vi "Project.vi"() -> ()   [LabVIEW 2015]
uses:
  <vilib>/Platform/TimedLoop/XDataNode/timing_clust.ctl
  <vilib>/Platform/TimedLoop/XDataNode/nitl_modes.ctl
  <vilib>/Platform/TimedLoop/XDataNode/wakeup.ctl
  <vilib>/DAQmx/read.llb/DAQmx Read (Counter DBL 1Chan 1Samp).vi
  <vilib>/DAQmx/read.llb/DAQmx Read (Digital Bool 1Line 1Point).vi
  <vilib>/DAQmx/write.llb/DAQmx Write (Analog DBL 1Chan 1Samp).vi
  <vilib>/DAQmx/read.llb/DAQmx Read (Analog 1D DBL NChan 1Samp).vi
  <vilib>/DAQmx/create/channels.llb/DAQmx Create Channel (AI-Voltage-Basic).vi
  <vilib>/DAQmx/create/channels.llb/DAQmx Create Channel (DI-Digital Input).vi
  <vilib>/DAQmx/create/channels.llb/DAQmx Create Channel (AO-Voltage-Basic).vi
  <vilib>/DAQmx/create/channels.llb/DAQmx Create Channel (CI-Count Edges).vi
  <vilib>/DAQmx/miscellaneous.llb/DAQmx Fill In Error Info.vi
  <vilib>/Analysis/3filter.llb/Butterworth Filter (DBL).vi
  <vilib>/Utility/file.llb/Write To Spreadsheet File (DBL).vi
  <vilib>/Platform/TimedLoop/XDataNode/XDataNode.xnode
  <vilib>/Platform/TimedLoop/XDataNode/XDNodeRunTimeDep.lvlib
  <vilib>/Analysis/NI_AALBase.lvlib
panel:
  out "Controller samp. time (s)":dbl
  out "Position Vs Time":cluster{dbl, "output":dbl}(graph)
  out "Force Vs Time":cluster{dbl, "output":dbl}(graph)
  out "Gripping Time":dbl format="%0.2f"
  out "Actual Force":dbl(slide) scale=0.0..20.0
  in  "Reset 2":bool
  in  "Desired Force":dbl(slide) min=0.0 max=13.5 scale=0.0..20.0 scale format="%#_3g"
  in  "Kd (force)":dbl=0.1 step=1.0
  in  "Ki (force)":dbl=0.5 step=2.0
  in  "Kp (force)":dbl=0.1 step=1.0
  in  "Kd (pos)":dbl=0.2 step=1.0
  in  "Ki (pos)":dbl=5.0 step=2.0
  in  "Kp (pos)":dbl=5.0 step=1.0
  out "Applied Motor Voltage":dbl
  out "Current Position":dbl(slide) scale=0.0..20.0
  out "Object Size":dbl(slide) scale=0.0..50.0
  out "Motor Position (deg.)":ext(knob) scale=0.0..360.0
  in  "Position Encoder":tag="Dev4/ctr0"
  out "Clockwise":bool
  in  "Optical Encoder":tag="Dev4/port0/line6"
  in  "Tachometer":tag="Dev4/ai4"
  in  "Current":tag="Dev4/ai0"
  in  "Voltage":tag="Dev4/ao0"
  in  "Reset":bool
  in  "Desired Position":dbl(slide) min=0.0 max=18.5 scale=0.0..20.0
  out "Motor & External Torque":cluster{dbl, dbl}(graph)
  out "Motor Acceleration (rad/s^2)":dbl(knob) scale=-50.0..50.0
  out "Motor Velocity (rad/s)":ext(knob) scale=-150.0..150.0
  out "Current Draw (amps)":dbl format="%#_2g"
  out "Current Draw":dbl(graph)
  out "Applied & Terminal Motor Voltage":cluster{dbl, "output":dbl}(graph)
  in  "File Path":path=path "\\\\uoa.auckland.ac.nz\\engdfs/home/nlob862/Desktop/705/dummy_stop_csv.csv"
  in  "?":bool
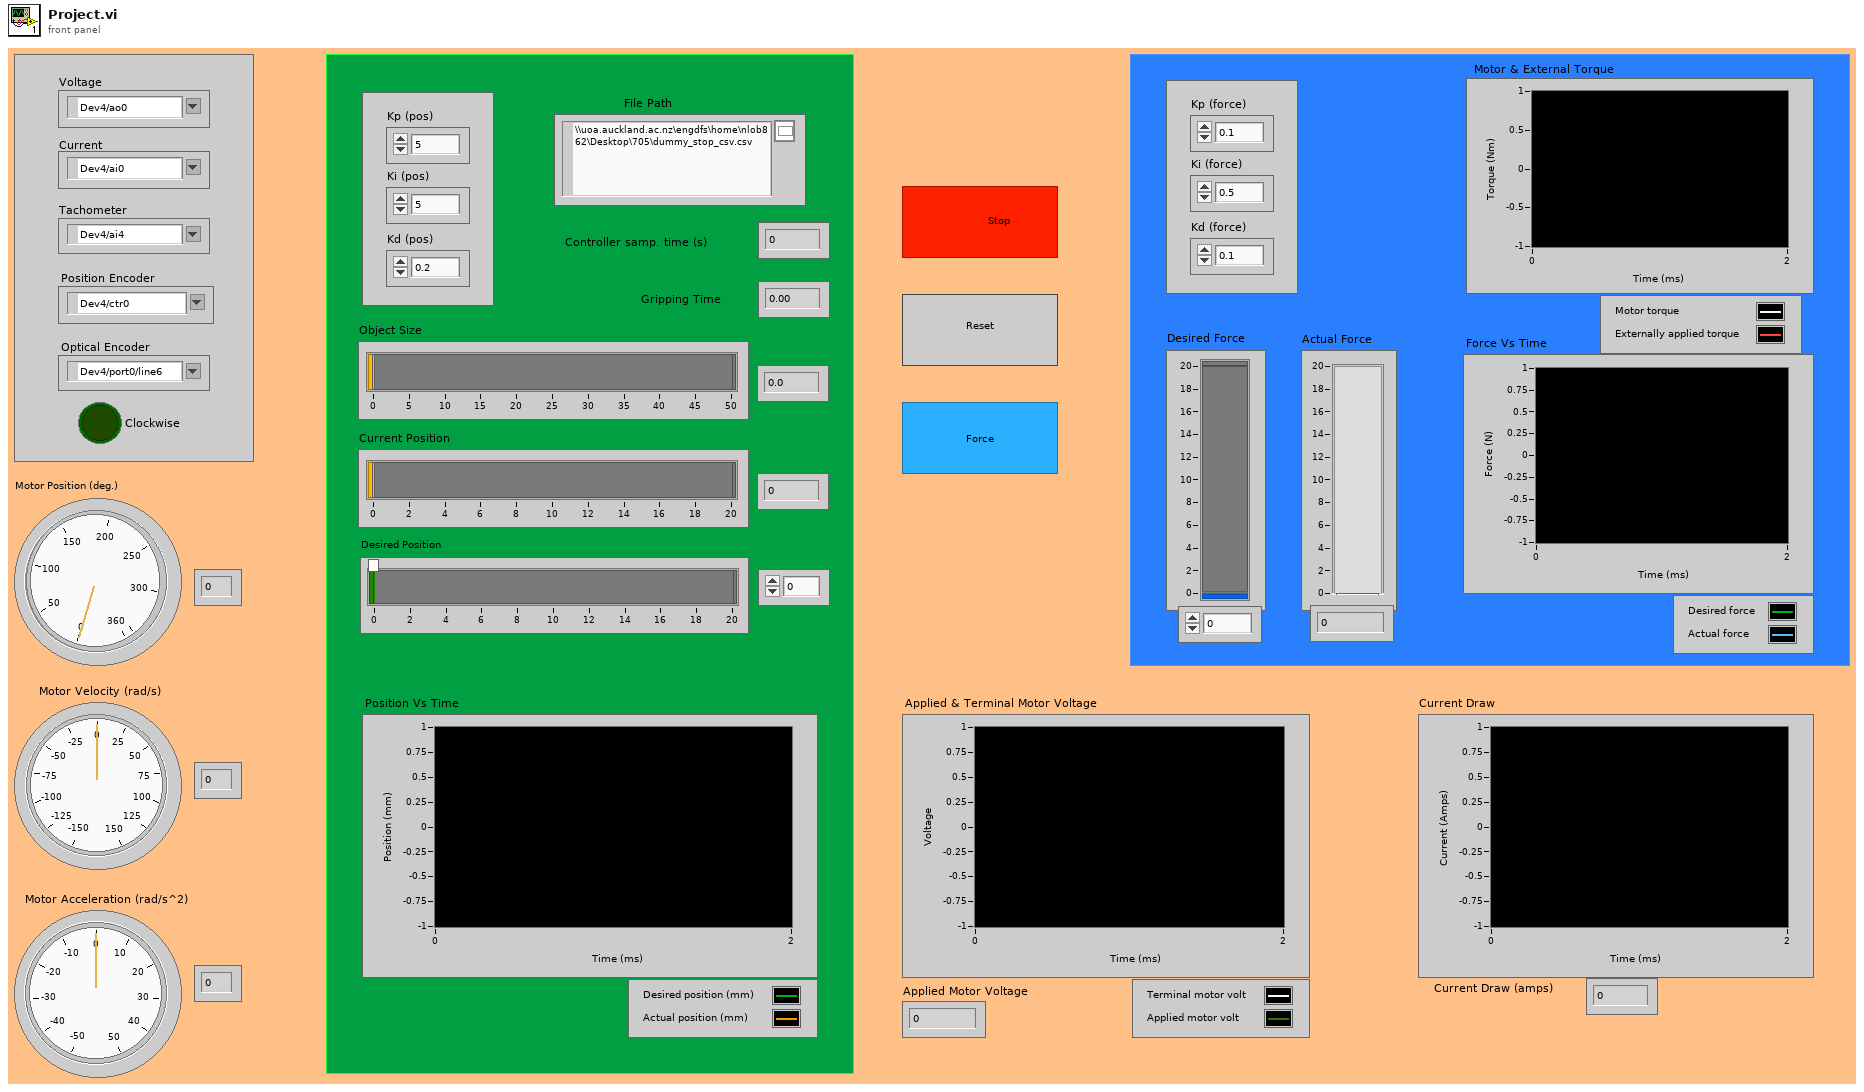
[diagram p1: front panel]
types:
  T1 = typedef "XDNodeRunTimeDep.lvlib/timing_clust.ctl" = cluster{"Expected End [f-1]":u64, "Actual End [f-1]":u64, "Finished Late? [f-1]":bool, "Expected End [i-1]":u64, "Actual End [i-1]":u64, "Finished Late? [i-1]":bool, "Expected Start [i]":u64, "Actual Start [i]":u64, "Expected Start [f]":u64, "Actual Start [f]":u64, "Source Name":string, "Structure Name":string, "Period":i64, "Deadline":i64, "Offset":i64, "Start":i64, "Priority":i32, "Timeout":i32, "Mode":T2, "Wakeup Reason":T3, "Error":errorcluster, "Source Type":string, "Secondary Source Type":string, "Global End Time":u64, "Global Start Time":u64, "Frame Duration":u64, "Iteration Duration":u64, "Assigned CPU":i32, "I/O Scan Engine Mode":u32}
  T2 = typedef "XDNodeRunTimeDep.lvlib/nitl_modes.ctl" = enum32{"No Change", "Process missed periods, maintain original phase", "Discard missed periods, maintain original phase", "Process missed periods, ignore original phase", "Discard missed periods, ignore original phase"}
  T3 = typedef "XDNodeRunTimeDep.lvlib/wakeup.ctl" = enum32{"Normal", "Aborted", "Asynchronous wakeup", "Timing source error", "Timed loop error", "Timeout"}
  T4 = cluster{"Desired Position":dbl, "Current Position":dbl}
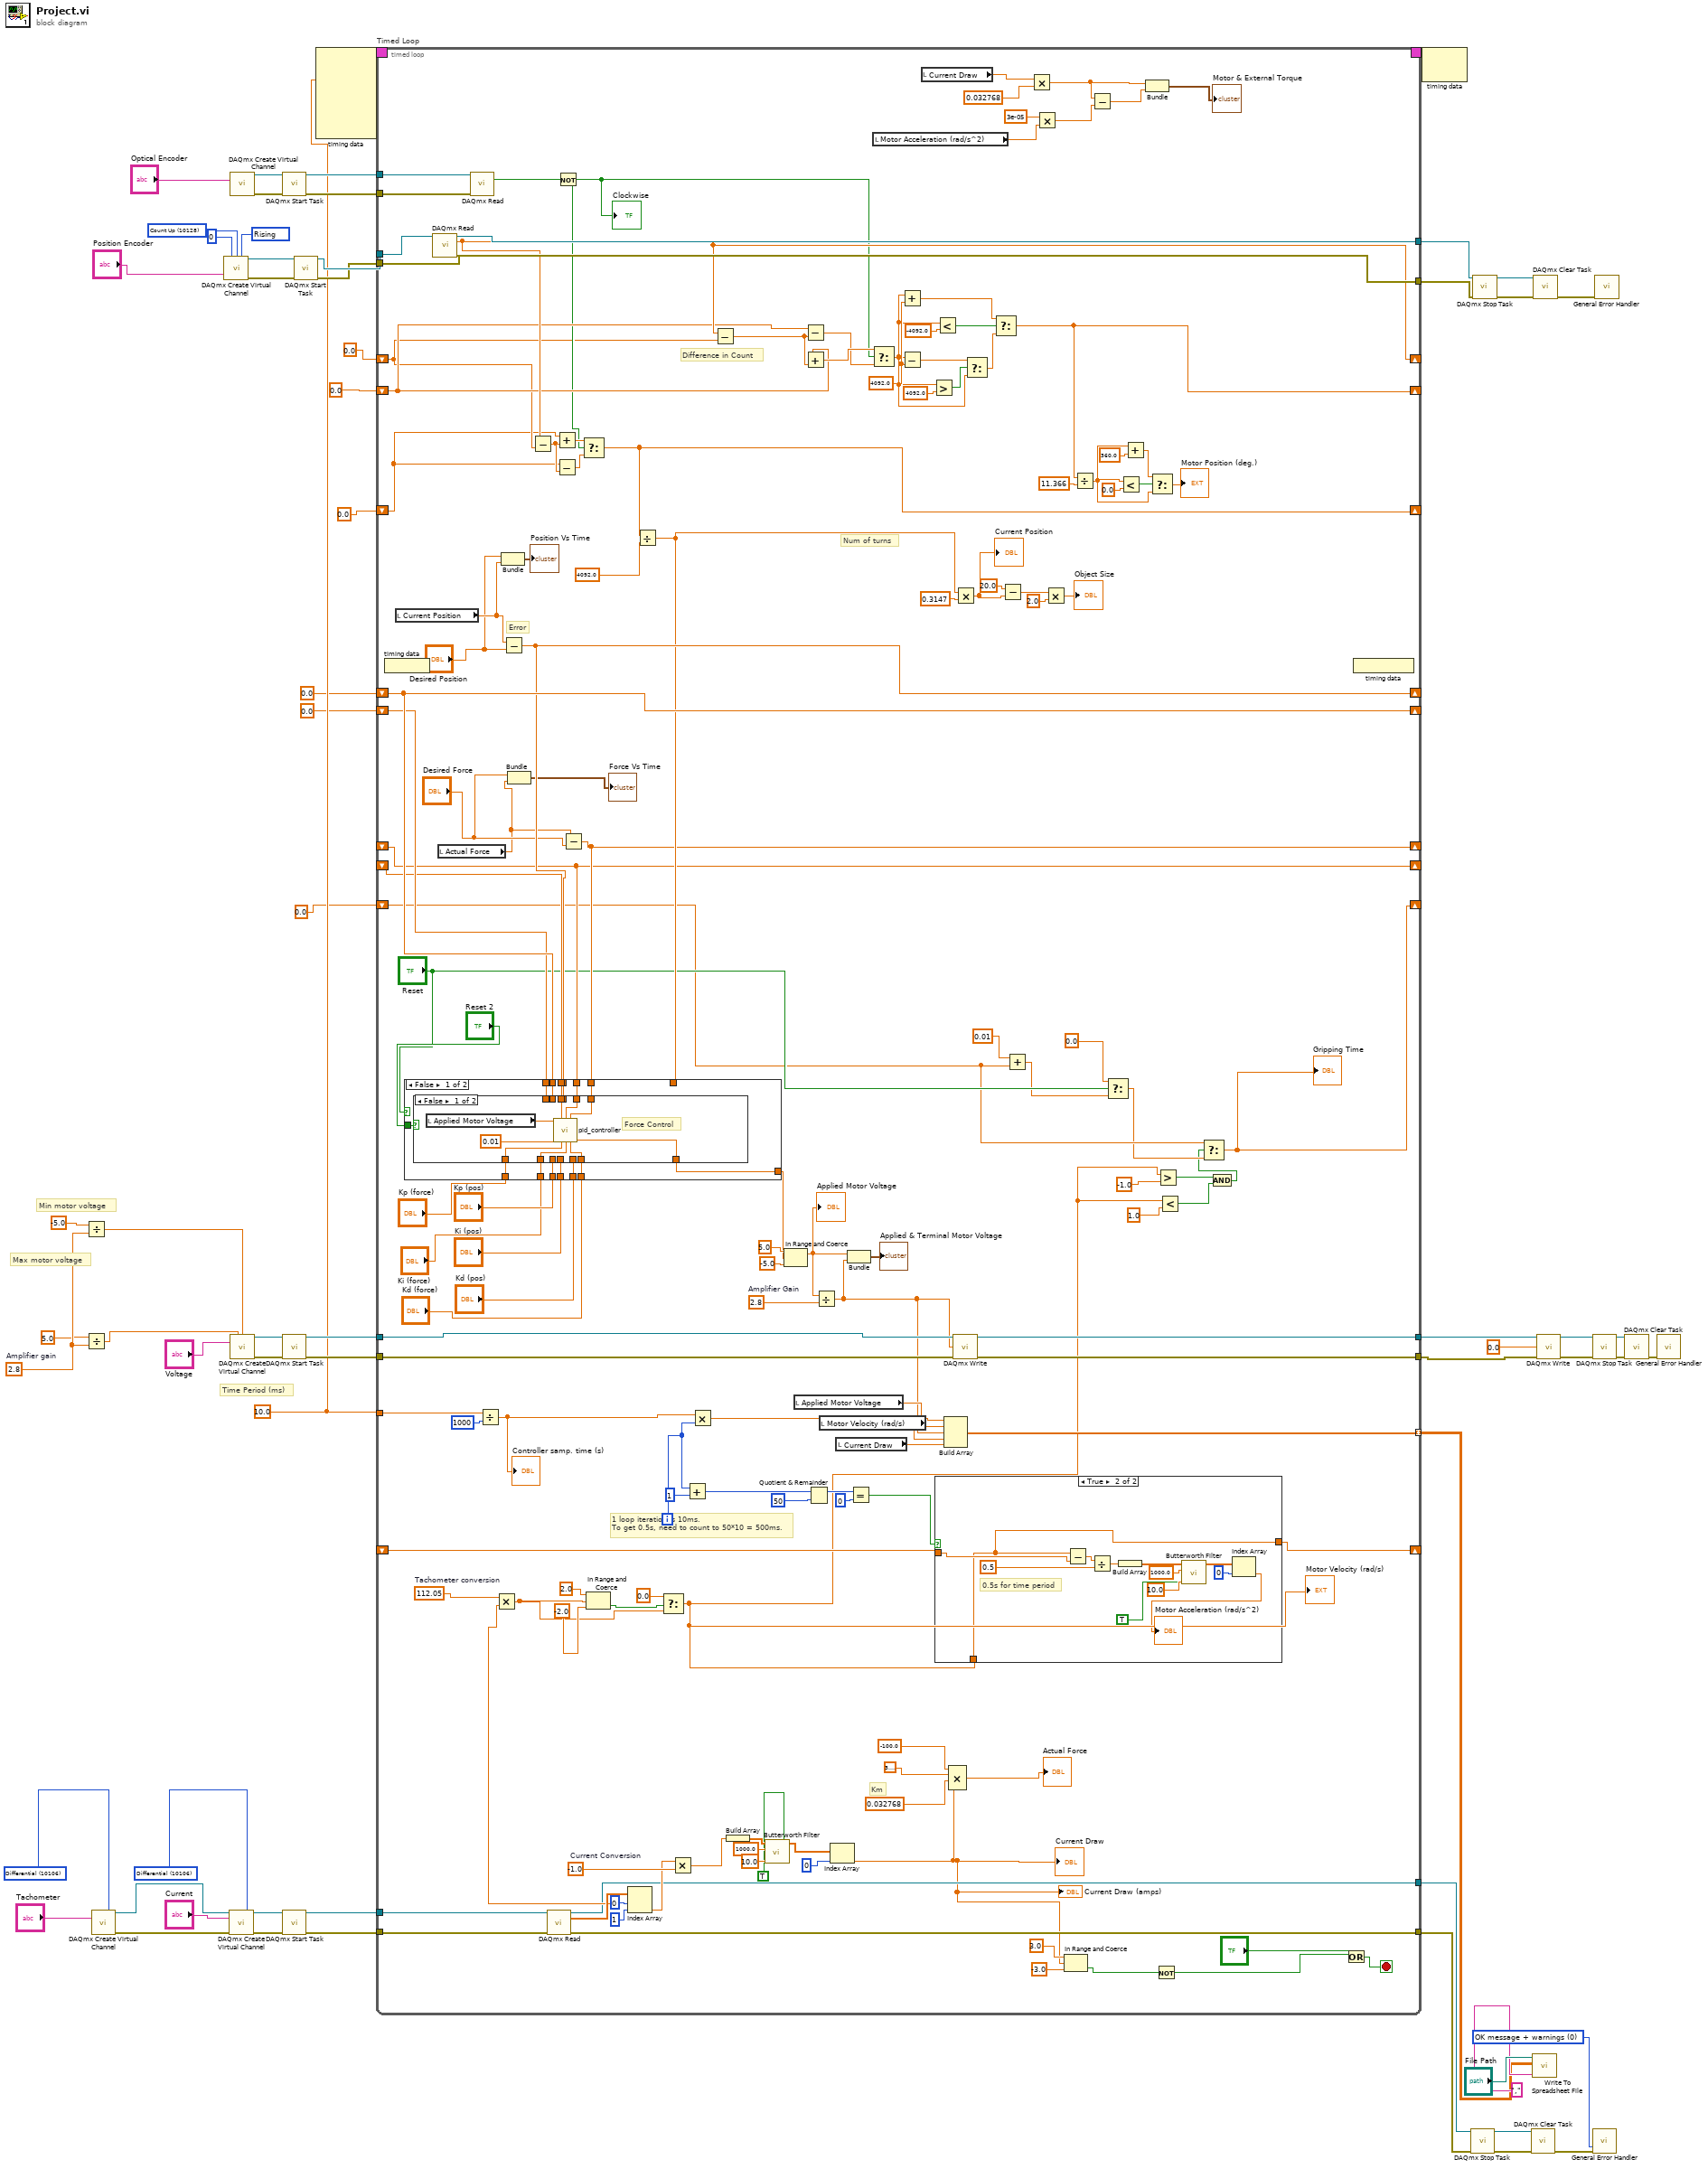
[diagram p0: block diagram]
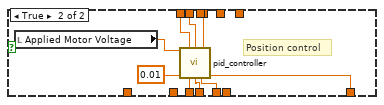
[diagram p2: hidden frame]
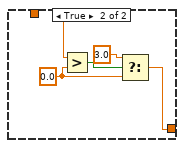
[diagram p3: hidden frame]
diagram:
  w4 = 10.0
  w8 = 10128 items=["Count Up"=10128, "Count Down"=10124, "Externally Controlled"=10326] ("count direction")
  w16 = 10280 items=["Rising"=10280, "Falling"=10171] ("edge")
  w31 = 10106 items=["Default"=-1, "RSE"=10083, "NRSE"=10078, "Differential"=10106, "Pseudodifferential"=12529] ("input terminal configuration")
  w32 = 10106 items=["Default"=-1, "RSE"=10083, "NRSE"=10078, "Differential"=10106, "Pseudodifferential"=12529] ("input terminal configuration")
  w44 = u16 0 items=["OK message + warnings"]
  w30 = 2.8  # Amplifier gain
  # "Time Period (ms)"
  # "Max motor voltage"
  # "Min motor voltage"
  n1 = Divide(x=-5.0, y=w30) -> (x/y=w49:dbl)
  n2 = Divide(x=5.0, y=w30) -> (x/y=w29:dbl)
  n3 = call-poly <vilib>:"DAQmx Create Virtual Channel.vi"("input terminal configuration"=w31, "physical channels"="Tachometer") -> ("task out"=w55:refnum<k21>, "error out"=w58:errorcluster)  [unwired: 12 in]
  n4 = call-poly <vilib>:"DAQmx Create Virtual Channel.vi"("initial count"=u32 0, "count direction"=w8, "edge"=w16, "counter"="Position Encoder") -> ("task out"=w20:refnum<k21>, "error out"=w19:errorcluster)  [unwired: 10 in]
  n5 = call-poly <vilib>:"DAQmx Create Virtual Channel.vi"("task in"=w55, "input terminal configuration"=w32, "physical channels"="Current", "error in"=w58) -> ("task out"=w56:refnum<k21>, "error out"=w57:errorcluster)  [unwired: 10 in]
  n6 = call-poly <vilib>:"DAQmx Create Virtual Channel.vi"("lines"="Optical Encoder") -> ("task out"=w27:refnum<k21>, "error out"=w25:errorcluster)  [unwired: 13 in]
  n7 = call-poly <vilib>:"DAQmx Create Virtual Channel.vi"("maximum value"=w29, "minimum value"=w49, "physical channels"="Voltage") -> ("task out"=w62:refnum<k21>, "error out"=w61:errorcluster)  [unwired: 11 in]
  n8 = call <vilib>:"DAQmx Start Task.vi"("task/channels in"=w27, "error in"=w25) -> ("task out"=w26:refnum<k21>, "error out"=w24:errorcluster)  [unwired: 12 in]
  n9 = call <vilib>:"DAQmx Start Task.vi"("task/channels in"=w62, "error in"=w61) -> ("task out"=w51:refnum<k21>, "error out"=w50:errorcluster)  [unwired: 12 in]
  n10 = call <vilib>:"DAQmx Start Task.vi"("task/channels in"=w56, "error in"=w57) -> ("task out"=w54:refnum<k21>, "error out"=w53:errorcluster)  [unwired: 12 in]
  n11 = call <vilib>:"DAQmx Start Task.vi"("task/channels in"=w20, "error in"=w19) -> ("task out"=w18:refnum<k21>, "error out"=w14:errorcluster)  [unwired: 12 in]
  n12 = node-c288(w4) -> (w64:T1)  [unwired: 5 in]
  n13 = timed-loop "Timed Loop" {
    timing: w64 -> [_]
    timing-out: [_] -> w63
    tunnel: w54 -> [w210]
    tunnel: w53 -> [w209]
    tunnel: w51 -> [w194]
    tunnel: w50 -> [w193]
    tunnel: [w197] -> w40
    tunnel: [w196] -> w39
    tunnel: w4 -> [w195]
    tunnel: [w191] -> w36
    tunnel: [w192] -> w38
    tunnel: [w199] -> w33 mode=indexing
    tunnel: w26 -> [w188]
    tunnel: w24 -> [w187]
    shift-right: [w182] -> _
    shift-left: _ -> [w183]
    tunnel: w18 -> [w169]
    tunnel: w14 -> [w168]
    tunnel: [w167] -> w10
    tunnel: [w166] -> w9
    shift-right: [w143] -> _
    shift-left: 0.0 -> [w139]
    shift-right: [w151] -> _
    shift-left: 0.0 -> [w142]
    shift-right: [w137] -> _
    shift-left: 0.0 -> [w138]
    shift-right: [w117] -> _
    shift-left: 0.0 -> [w122]
    shift-right: [w122] -> _
    shift-left: 0.0 -> [w121]
    shift-right: [w111] -> _
    shift-left: _ -> [w110]
    shift-right: [w110] -> _
    shift-left: _ -> [w109]
    shift-right: [w96] -> _
    shift-left: 0.0 -> [w97]
    i -> [w185]
    stop <- w76 stop-if-true
    w156 = 4092.0
    w208 = -1.0  # Current Conversion
    w207 = 112.05  # Tachometer conversion
    w198 = 2.8  # Amplifier Gain
    # "Num of turns"
    # "Km"
    # "Error"
    # "Difference in Count"
    # "1 loop iteration is 10ms.\nTo get 0.5s, need to count to 50*10 = 500ms."
    n14 = node-c288() -> ()  [unwired: 1 in]
    n15 = local read "Current Position"() -> (w86:dbl)
    n16 = call-poly <vilib>:"DAQmx Read.vi"("task/channels in"=w169, "error in"=w168) -> ("task out"=w167:refnum<k21>, "data"=w143:dbl, "error out"=w166:errorcluster)  [unwired: 11 in]
    n17 = local read "Actual Force"() -> (w65:dbl)
    n18 = call-poly <vilib>:"DAQmx Read.vi"("task/channels in"=w188, "error in"=w187) -> ("data"=w186:bool)  [unwired: 11 in, 2 out]
    n19 = Divide(x=w195, y=1000) -> (x/y=w126:dbl)
    "Controller samp. time (s)" <- w126
    n20 = Bundle("Desired Position"="Desired Position", "Current Position"=w86) -> (→"Position Vs Time":T4)  [unwired: 1 in]
    n21 = Subtract(x=w86, y="Desired Position") -> (x-y=w117:dbl)
    n22 = Bundle("Desired Force"="Desired Force", "Actual Force"=w65) -> (→"Force Vs Time":cluster{"Desired Force":dbl, "Actual Force":dbl})  [unwired: 1 in]
    n23 = Subtract(x=w143, y=w139) -> (x-y=w141:dbl)
    n24 = call-poly <vilib>:"DAQmx Read.vi"("task/channels in"=w210, "error in"=w209) -> ("task out"=w196:refnum<k21>, "data"=w206:dbl[], "error out"=w197:errorcluster)  [unwired: 11 in]
    n25 = Add(x=w138, y=w141) -> (x+y=w145:dbl)
    n26 = Subtract(x=w138, y=w141) -> (x-y=w144:dbl)
    n27 = Not(x=w186) -> (.not. x?=w140:bool)
    "Clockwise" <- w140
    n28 = Subtract(x=w65, y="Desired Force") -> (x-y=w111:dbl)
    n29 = Select(t=w145, s=w140, f=w144) -> (s? t:f=w137:dbl)
    n30 = Index Array(array=w206, index #1=0, index #2=1) -> (element #1=w203:dbl, element #2=w202:dbl)
    n31 = Multiply(x=w207, y=w203) -> (x*y=w172:dbl)
    n32 = In Range and Coerce(upper limit=2.0, x=w172, lower limit=-2.0) -> (In Range?=w174:bool)  [unwired: 1 out]
    n33 = Divide(x=w137, y=4092.0) -> (x/y=w116:dbl)
    n34 = case shown="False" "Reset" {
      tunnel: w116 -> [_ w244]
      tunnel: [w218 w243] -> w123
      tunnel: w117 -> [w222 _]
      tunnel: w122 -> [w223 _]
      tunnel: w121 -> [w224 _]
      tunnel: "Kp (pos)" -> [w221 _]
      tunnel: "Ki (pos)" -> [w220 _]
      tunnel: "Kd (pos)" -> [w219 _]
      tunnel: "Reset 2" -> [w217 _]
      tunnel: "Kp (force)" -> [w216 _]
      tunnel: "Ki (force)" -> [w215 _]
      tunnel: "Kd (force)" -> [w214 _]
      tunnel: w111 -> [w213 _]
      tunnel: w110 -> [w212 _]
      tunnel: w109 -> [w211 _]
      frame False {
        n35 = case shown="False" w217 {
          tunnel: w224 -> [_ w242]
          tunnel: w223 -> [_ w241]
          tunnel: w222 -> [_ w240]
          tunnel: w221 -> [_ w237]
          tunnel: w220 -> [_ w236]
          tunnel: w219 -> [_ w235]
          tunnel: [w225 w234] -> w218
          tunnel: w216 -> [w231 _]
          tunnel: w215 -> [w230 _]
          tunnel: w214 -> [w229 _]
          tunnel: w213 -> [w228 _]
          tunnel: w212 -> [w227 _]
          tunnel: w211 -> [w226 _]
          frame False {
            # "Force Control"
            n36 = local read "Applied Motor Voltage"() -> (w232:dbl)
            n37 = call "pid_controller.vi"("Motor Voltage 1 Sample Ago"=w232, "Error 2 Samples Ago"=w226, "Error 1 Sample Ago"=w227, "Error (Current)"=w228, "Time (dt)"=0.01, "Kp"=w231, "Ki"=w230, "Kd"=w229) -> ("Motor Voltage for Next Sample"=w225:dbl)  [unwired: 7 in]
          }
          frame True {
            # "Position control"
            n38 = local read "Applied Motor Voltage"() -> (w239:dbl)
            n39 = call "pid_controller.vi"("Motor Voltage 1 Sample Ago"=w239, "Error 2 Samples Ago"=w242, "Error 1 Sample Ago"=w241, "Error (Current)"=w240, "Time (dt)"=0.01, "Kp"=w237, "Ki"=w236, "Kd"=w235) -> ("Motor Voltage for Next Sample"=w234:dbl)  [unwired: 7 in]
          }
        }
      }
      frame True {
        w245 = 0.0
        n40 = Greater?(x=w244, y=w245) -> (0:w246:bool)
        n41 = Select(t=3.0, s=w246, f=w245) -> (s? t:f=w243:dbl)
      }
    }
    n42 = Select(t=0.0, s=w174, f=w172) -> (s? t:f=w92:dbl)
    "Motor Velocity (rad/s)" <- w92
    n43 = Multiply(x=w202, y=w208) -> (x*y=w80:dbl)
    n44 = Add(x=w185, y=1) -> (x+y=w179:i32)
    n45 = Multiply(x=w126, y=w185) -> (x*y=w200:dbl)
    n46 = Subtract(x=w143, y=w139) -> (x-y=w165:dbl)
    n47 = Build Array(w80) -> (w103:dbl[])
    n48 = call-poly <vilib>:"Butterworth Filter.vi"("init/cont (init:F)"=TRUE, "low cutoff freq: fl"=10.0, "sampling freq: fs"=1000.0, "X"=w103) -> ("Filtered X"=w74:dbl[])  [unwired: 4 in, 1 out]
    n49 = In Range and Coerce(upper limit=5.0, x=w123, lower limit=-5.0 ("upper limit")) -> (coerced(x)=w108:dbl)  [unwired: 1 out]
    "Applied Motor Voltage" <- w108
    n50 = local read "Applied Motor Voltage"() -> (w129:dbl)
    n51 = Subtract(x=w142, y=w165) -> (x-y=w163:dbl)
    n52 = Add(x=w142, y=w165) -> (x+y=w164:dbl)
    n53 = Quotient & Remainder(x=w179, y=50) -> (x-y*floor(x/y)=w178:i32)  [unwired: 1 out]
    n54 = Divide(x=w108, y=w198) -> (x/y=w125:dbl)
    n55 = local read "Motor Velocity (rad/s)"() -> (w190:ext)
    n56 = Index Array(array=w74, index=0) -> (element=w73:dbl)
    "Current Draw" <- w73
    "Current Draw (amps)" <- w73
    n57 = local read "Current Draw"() -> (w189:dbl)
    n58 = Bundle("upper limit"=w108, w125) -> (→"Applied & Terminal Motor Voltage":cluster{"upper limit":dbl, dbl})  [unwired: 1 in]
    n59 = Equal?(x=w178, y=0) -> (x = y?=w184:bool)
    n60 = Select(t=w164, s=w140, f=w163) -> (s? t:f=w146:dbl)
    n61 = local read "Motor Acceleration (rad/s^2)"() -> (w67:dbl)
    n62 = Add(x=w146, y=w156) -> (x+y=w155:dbl)
    n63 = Subtract(x=w146, y=w156) -> (x-y=w159:dbl)
    n64 = local read "Current Draw"() -> (w171:dbl)
    n65 = Greater?(x=w146, y=4092.0) -> (0:w160:bool)
    n66 = case shown="True" w184 {
      tunnel: w92 -> [_ w259]
      tunnel: w183 -> [w248 w260]
      tunnel: [w248 w259] -> w182
      frame False {
      }
      frame True {
        # "0.5s for time period"
        n67 = Subtract(x=w259, y=w260) -> (x-y=w258:dbl)
        n68 = Divide(x=w258, y=0.5) -> (x/y=w250:dbl)
        n69 = Build Array(w250) -> (w254:dbl[])
        n70 = call-poly <vilib>:"Butterworth Filter.vi"("init/cont (init:F)"=TRUE, "low cutoff freq: fl"=10.0, "sampling freq: fs"=1000.0, "X"=w254) -> ("Filtered X"=w251:dbl[])  [unwired: 4 in, 1 out]
        n71 = Index Array(array=w251, index=0) -> (element=→"Motor Acceleration (rad/s^2)":dbl)
      }
    }
    n72 = Less?(x=w146, y=-4092.0) -> (x < y?=w157:bool)
    n73 = Build Array(w200, w129, w125, w190, w189) -> (w199:ext[])
    n74 = Compound Arithmetic op=MULTIPLY(-100.0 ("x"), 3.141592653589793, 0.032768 ("x"), w73) -> (→"Actual Force":dbl)
    n75 = call-poly <vilib>:"DAQmx Write.vi"("task/channels in"=w194, "data"=w125, "error in"=w193) -> ("task out"=w191:refnum<k21>, "error out"=w192:errorcluster)  [unwired: 10 in, 1 out]
    n76 = Multiply(x=w116, y=0.3147) -> (x*y=w130:dbl)
    "Current Position" <- w130
    n77 = Select(t=w159, s=w160, f=w146) -> (s? t:f=w158:dbl)
    n78 = Select(t=w155, s=w157, f=w158) -> (s? t:f=w151:dbl)
    n79 = Subtract(x=20.0 ("y"), y=w130) -> (x-y=w134:dbl)
    n80 = Add(x=0.01 ("y"), y=w97) -> (x+y=w100:dbl)
    n81 = Multiply(x=w171, y=0.032768) -> (x*y=w71:dbl)
    n82 = Multiply(x=3e-05, y=w67) -> (x*y=w69:dbl)
    n83 = Multiply(x=w134, y=2.0) -> (x*y=→"Object Size":dbl)
    n84 = In Range and Coerce(upper limit=3.0, x=w73, lower limit=-3.0) -> (In Range?=w79:bool)  [unwired: 1 out]
    n85 = Divide(x=w151, y=11.366) -> (x/y=w147:dbl)
    n86 = Subtract(x=w71, y=w69) -> (x-y=w70:dbl)
    n87 = Select(t=0.0 ("y"), s="Reset", f=w100) -> (s? t:f=w95:dbl)
    n88 = Less?(x=w147, y=0.0) -> (x < y?=w152:bool)
    n89 = Add(x=w147, y=360.0) -> (x+y=w149:dbl)
    n90 = Bundle(w71, w70) -> (→"Motor & External Torque":cluster{dbl, dbl})  [unwired: 1 in]
    n91 = Select(t=w149, s=w152, f=w147) -> (s? t:f=→"Motor Position (deg.)":dbl)
    n92 = Not(x=w79) -> (.not. x?=w77:bool)
    n93 = Greater?(x=w92, y=-1.0) -> (0:w91:bool)
    n94 = Less?(x=w92, y=1.0) -> (x < y?=w94:bool)
    n95 = And(x=w91, y=w94) -> (x .and. y?=w90:bool)
    n96 = Select(t=w97, s=w90, f=w95) -> (s? t:f=w96:dbl)
    "Gripping Time" <- w96
    n97 = Or(x=w77, y="?") -> (x .or. y?=w76:bool)
    n98 = node-c288() -> ()  [unwired: 1 out]
  }
  n99 = node-c288(w63) -> ()  [unwired: 1 out]
  n100 = call <vilib>:"DAQmx Stop Task.vi"("task/channels in"=w39, "error in"=w40) -> ("task out"=w42:refnum<k21>, "error out"=w43:errorcluster)  [unwired: 12 in]
  n101 = call <vilib>:"DAQmx Stop Task.vi"("task/channels in"=w10, "error in"=w9) -> ("task out"=w12:refnum<k21>, "error out"=w13:errorcluster)  [unwired: 12 in]
  n102 = call <vilib>:"DAQmx Clear Task.vi"("task in"=w42, "error in"=w43) -> ("error out"=w41:errorcluster)  [unwired: 13 in]
  n103 = call-poly <vilib>:"Write To Spreadsheet File.vi"("delimiter (\\t)"=",", "2D data"=w33, "file path (dialog if empty)"="File Path") -> ()  [unwired: 5 in, 1 out]
  n104 = call <vilib>:"DAQmx Clear Task.vi"("task in"=w12, "error in"=w13) -> ("error out"=w11:errorcluster)  [unwired: 13 in]
  n105 = call-poly <vilib>:"DAQmx Write.vi"("task/channels in"=w36, "data"=0.0, "error in"=w38) -> ("task out"=w37:refnum<k21>, "error out"=w46:errorcluster)  [unwired: 10 in, 1 out]
  n106 = call <vilib>:"DAQmx Stop Task.vi"("task/channels in"=w37, "error in"=w46) -> ("task out"=w48:refnum<k21>, "error out"=w47:errorcluster)  [unwired: 12 in]
  n107 = call <vilib>:"General Error Handler.vi"("type of dialog (OK msg:1)"=w44, "error in (no error)"=w41) -> ()  [unwired: 9 in, 5 out]
  n108 = call <vilib>:"General Error Handler.vi"("error in (no error)"=w11) -> ()  [unwired: 10 in, 5 out]
  n109 = call <vilib>:"DAQmx Clear Task.vi"("task in"=w48, "error in"=w47) -> ("error out"=w45:errorcluster)  [unwired: 13 in]
  n110 = call <vilib>:"General Error Handler.vi"("error in (no error)"=w45) -> ()  [unwired: 10 in, 5 out]
